vi "GetRelativeAngle.vi"(8 "error in (no error)":errorcluster, 10 "Boat Angle (Deg.)":dbl, 11 "Angle in":refnum<class "Angle.lvclass">) -> (0 "error out":errorcluster, 2 "Relative Angle":dbl)   [LabVIEW 2011, in "Angle.lvclass"]
uses:
  Angle.lvclass
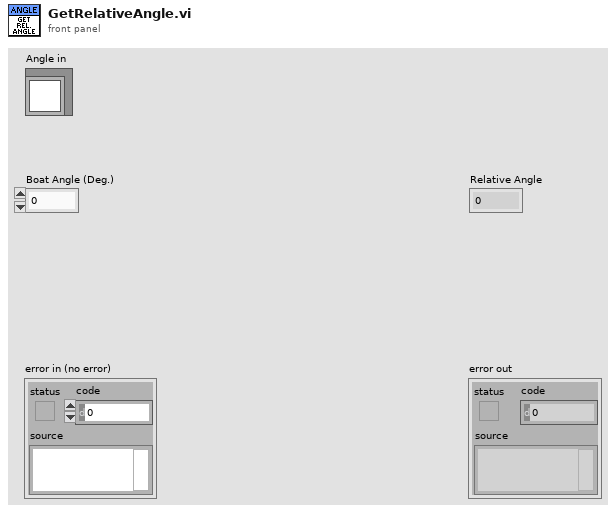
[diagram p1: front panel]
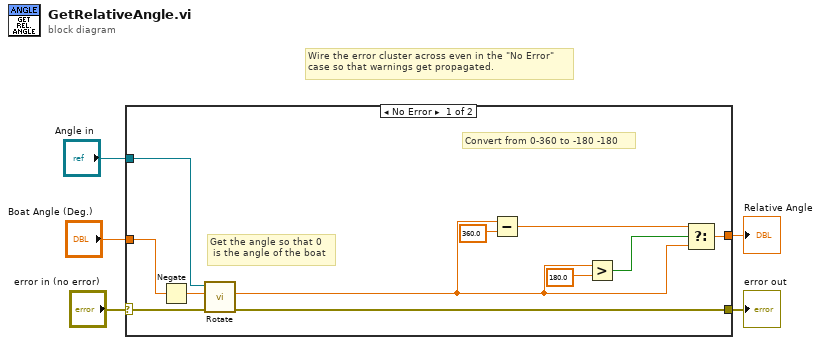
[diagram p0: block diagram]
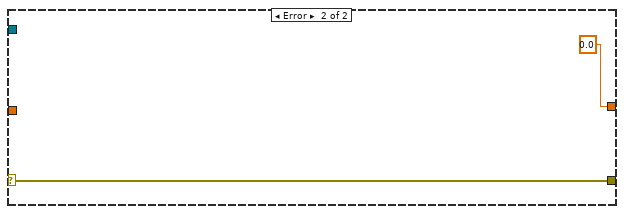
[diagram p2: hidden frame]
diagram:
  # "Wire the error cluster across even in the \"No Error\"\ncase so that warnings get propagated."
  n1 = case shown="No Error" "error in (no error)" {
    selector: "error in (no error)" -> [w16 w18]
    tunnel: [w15 w18] -> w4
    tunnel: "Angle in" -> [w14 _]
    tunnel: [w8 0.0 ("New Angle")] -> w2
    tunnel: "Boat Angle (Deg.)" -> [w6 _]
    frame No Error {
      # "Convert from 0-360 to -180 -180"
      # "Get the angle so that 0\n is the angle of the boat"
      n2 = Negate(x=w6) -> (-x=w7:dbl)
      n3 = call "Rotate.vi"("error in (no error)"=w16, "Rotation Angle (Deg.)"=w7, "Angle in"=w14) -> ("error out"=w15:errorcluster, "New Angle"=w9:dbl)  [unwired: 6 in, 1 out]
      n4 = Subtract(x=w9, y=360.0) -> (x-y=w11:dbl)
      n5 = Greater?(x=w9, y=180.0) -> (0:w13:bool)
      n6 = Select(t=w11, s=w13, f=w9) -> (s? t:f=w8:dbl)
    }
    frame Error {
    }
  }
  "error out" <- w4
  "Relative Angle" <- w2
